vi "SaveLoadPreview-main.vi"(6 "error in":errorcluster, 10 "Prev-Save-Load":T1) -> (4 "error out 3":errorcluster)   [LabVIEW 2016, in "SaveLoad.lvlib"]
doc: "Takes a vi and saves or loads set values depending on which cluster value is chosen"
uses:
  SaveLoad.lvlib
  saveloadprev.ctl
  Beamline sections/High Energy End/High energy.lvlib
  Beamline sections/R30/R30.lvlib
  Beamline sections/Transmission/Transmission.lvlib
  Beamline sections/Low Energy End/Low energy.lvlib
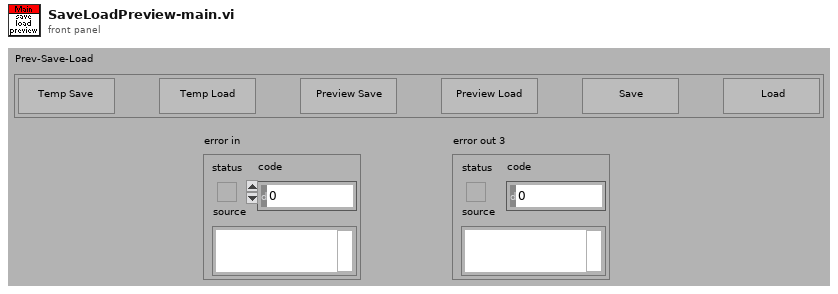
[diagram p1: front panel]
types:
  T1 = typedef "saveloadprev.ctl" = cluster{"Temp Save":bool, "Temp Load":bool, "Save":bool, "Load":bool, "Preview Save":bool, "Preview Load":bool}
  T2 = enum16{"open", "replace", "create", "open or create", "replace or create", "replace or create with confirmation"}
  T3 = typedef "prev-save-load-enum.ctl" = enum16{"Temp Save", "Temp Load", "Save", "Load", "Preview Save", "Preview Load"}
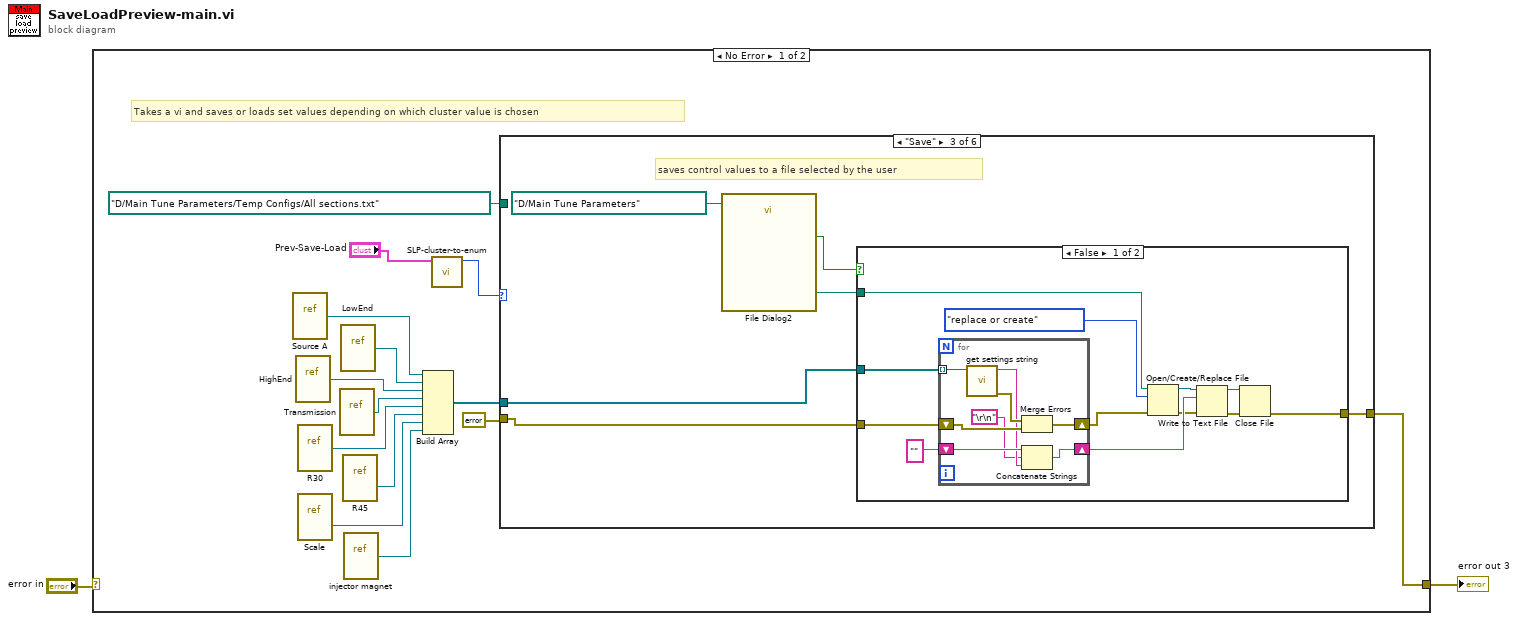
[diagram p0: block diagram]
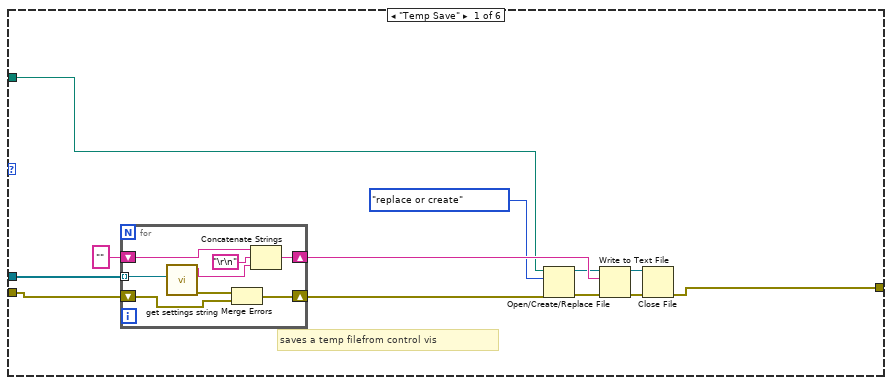
[diagram p2: hidden frame]
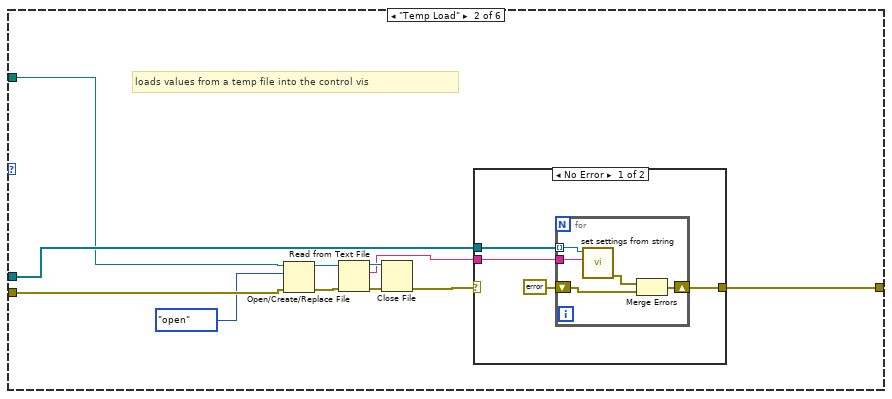
[diagram p3: hidden frame]
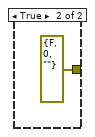
[diagram p5: hidden frame]
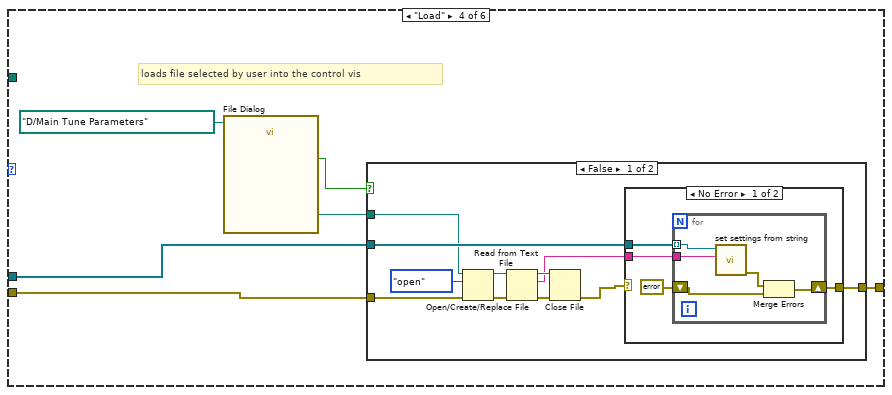
[diagram p6: hidden frame]
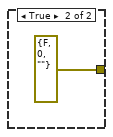
[diagram p8: hidden frame]
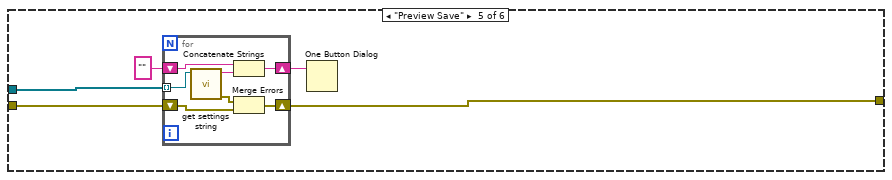
[diagram p9: hidden frame]
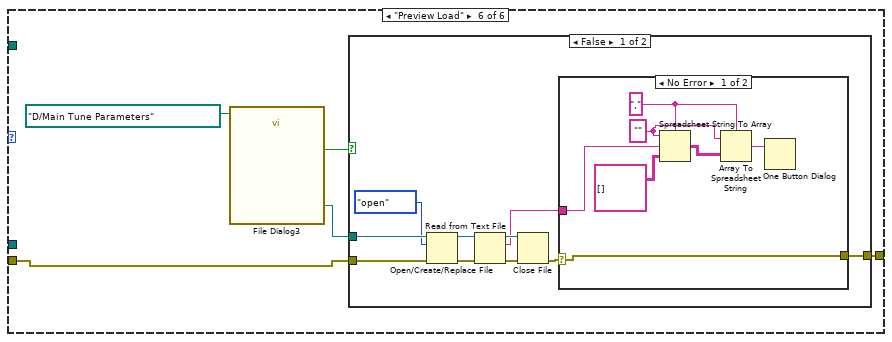
[diagram p10: hidden frame]
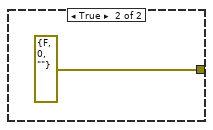
[diagram p12: hidden frame]
diagram:
  n1 = case shown="No Error" "error in" {
    selector: "error in" -> [_ w149]
    tunnel: [w16 w149] -> w2
    frame No Error {
      # "Takes a vi and saves or loads set values depending on which cluster value is chosen"
      n2 = vi-ref "Source A.vi"() -> (w10:refnum<vi>)
      n3 = vi-ref "HighEnd.vi"() -> (w14:refnum<vi>)
      n4 = vi-ref "R30.vi"() -> (w13:refnum<vi>)
      n5 = vi-ref "Scale.vi"() -> (w9:refnum<vi>)
      n6 = vi-ref "Transmission.vi"() -> (w15:refnum<vi>)
      n7 = vi-ref "LowEnd.vi"() -> (w11:refnum<vi>)
      n8 = vi-ref "R45.vi"() -> (w12:refnum<vi>)
      n9 = vi-ref "injector magnet.vi"() -> (w8:refnum<vi>)
      n10 = Build Array(w10, w11, w14, w15, w13, w12, w9, w8) -> (w7:refnum<vi>[])
      n11 = call "SLP-cluster-to-enum.vi"("Prev-Save-Load"="Prev-Save-Load") -> ("Prev-Save-Load enum"=w5:T3)  [unwired: 10 in]
      n12 = case shown="\"Save\"" w5 {
        tunnel: errorcluster {"status"=FALSE, "code"=0, "source"=""} ("error IO") -> [w17 w39 w62 w88 w113 w126]
        tunnel: [w24 w43 w61 w89 w114 w129] -> w16
        tunnel: w7 -> [w22 w45 w63 w90 w117 _]
        tunnel: path "D:/Main Tune Parameters/Temp Configs/All sections.txt" ("file path (use dialog)") -> [w20 w40 _ _ _ _]
        frame "Temp Save" {
          # "saves a temp filefrom control vis"
          n13 = for {
            shift-right: [w35] -> w28
            shift-left: "" -> [w34]
            tunnel: w22 -> [w33] mode=indexing
            shift-right: [w30] -> w23
            shift-left: w17 -> [w29]
            n14 = call "get settings string.vi"("VI in"=w33) -> ("error out"=w32:errorcluster, "Settings string"=w31:string)  [unwired: 9 in]
            n15 = Merge Errors(w32, w29) -> (w30:errorcluster)
            n16 = Concatenate Strings(w34, "\r\n", w31) -> (w35:string)
          }
          n17 = Open/Create/Replace File(file path (use dialog)=w20, error in=w23, operation (0:open)=T2."replace or create") -> (refnum out=w19:refnum<file>, error out=w21:errorcluster)  [unwired: 3 in, 1 out]
          n18 = Write to Text File(file (use dialog)=w19, text=w28, error in=w21) -> (refnum out=w26:refnum<file>, error out=w25:errorcluster)  [unwired: 1 in, 1 out]
          n19 = Close File(refnum=w26, error in=w25) -> (error out=w24:errorcluster)  [unwired: 1 out]
        }
        frame "Temp Load" {
          # "loads values from a temp file into the control vis"
          n20 = Open/Create/Replace File(file path (use dialog)=w40, error in=w39, operation (0:open)=T2."open") -> (refnum out=w41:refnum<file>, error out=w42:errorcluster)  [unwired: 3 in, 1 out]
          n21 = Read from Text File(file (use dialog)=w41, error in=w42) -> (refnum out=w47:refnum<file>, text=w44:string, error out=w46:errorcluster)  [unwired: 3 out]
          n22 = Close File(refnum=w47, error in=w46) -> (error out=w37:errorcluster)  [unwired: 1 out]
          n23 = case shown="No Error" w37 {
            selector: w37 -> [_ w57]
            tunnel: w45 -> [w51 _]
            tunnel: w44 -> [w50 _]
            tunnel: [w49 w57] -> w43
            frame No Error {
              n24 = for {
                tunnel: w51 -> [w55] mode=indexing
                tunnel: w50 -> [w56]
                shift-right: [w54] -> w49
                shift-left: errorcluster {"status"=FALSE, "code"=0, "source"=""} ("error IO") -> [w52]
                n25 = call "set settings from string.vi"("String"=w56, "VI in"=w55) -> ("error out"=w53:errorcluster)  [unwired: 9 in]
                n26 = Merge Errors(w53, w52) -> (w54:errorcluster)
              }
            }
            frame Error {
            }
          }
        }
        frame "Save" {
          # "saves control values to a file selected by the user"
          n27 = call "File Dialog2"("start path"=path "D:/Main Tune Parameters") -> ("selected path"=w59:path, "cancelled"=w58:bool)  [unwired: 11 in, 2 out]
          n28 = case shown="False" w58 {
            tunnel: w63 -> [w72 _]
            tunnel: w62 -> [w71 _]
            tunnel: [w64 errorcluster {"status"=FALSE, "code"=0, "source"=""} ("error out")] -> w61
            tunnel: w59 -> [w65 _]
            frame False {
              n29 = for {
                tunnel: w72 -> [w83] mode=indexing
                shift-right: [w81] -> w66
                shift-left: w71 -> [w80]
                shift-right: [w79] -> w70
                shift-left: "" -> [w78]
                n30 = call "get settings string.vi"("VI in"=w83) -> ("error out"=w82:errorcluster, "Settings string"=w77:string)  [unwired: 9 in]
                n31 = Merge Errors(w82, w80) -> (w81:errorcluster)
                n32 = Concatenate Strings(w78, "\r\n", w77) -> (w79:string)
              }
              n33 = Open/Create/Replace File(file path (use dialog)=w65, error in=w66, operation (0:open)=T2."replace or create") -> (refnum out=w68:refnum<file>, error out=w67:errorcluster)  [unwired: 1 in, 3 out]
              n34 = Write to Text File(file (use dialog)=w68, text=w70, error in=w67) -> (refnum out=w75:refnum<file>, error out=w74:errorcluster)  [unwired: 1 in, 1 out]
              n35 = Close File(refnum=w75, error in=w74) -> (error out=w64:errorcluster)  [unwired: 1 out]
            }
            frame True {
            }
          }
        }
        frame "Load" {
          # "loads file selected by user into the control vis"
          n36 = call "File Dialog"("start path"=path "D:/Main Tune Parameters") -> ("selected path"=w87:path, "cancelled"=w85:bool)  [unwired: 11 in, 2 out]
          n37 = case shown="False" w85 {
            tunnel: w90 -> [w99 _]
            tunnel: [w97 errorcluster {"status"=FALSE, "code"=0, "source"=""} ("error out")] -> w89
            tunnel: w88 -> [w96 _]
            tunnel: w87 -> [w92 _]
            frame False {
              n38 = Open/Create/Replace File(file path (use dialog)=w92, error in=w96, operation (0:open)=T2."open") -> (refnum out=w94:refnum<file>, error out=w95:errorcluster)  [unwired: 3 in, 1 out]
              n39 = Read from Text File(file (use dialog)=w94, error in=w95) -> (refnum out=w100:refnum<file>, text=w98:string, error out=w101:errorcluster)  [unwired: 3 out]
              n40 = Close File(refnum=w100, error in=w101) -> (error out=w91:errorcluster)  [unwired: 1 out]
              n41 = case shown="No Error" w91 {
                selector: w91 -> [_ w111]
                tunnel: w99 -> [w105 _]
                tunnel: w98 -> [w104 _]
                tunnel: [w103 w111] -> w97
                frame No Error {
                  n42 = for {
                    tunnel: w105 -> [w109] mode=indexing
                    tunnel: w104 -> [w110]
                    shift-right: [w108] -> w103
                    shift-left: errorcluster {"status"=FALSE, "code"=0, "source"=""} ("error IO") -> [w106]
                    n43 = call "set settings from string.vi"("String"=w110, "VI in"=w109) -> ("error out"=w107:errorcluster)  [unwired: 9 in]
                    n44 = Merge Errors(w107, w106) -> (w108:errorcluster)
                  }
                }
                frame Error {
                }
              }
            }
            frame True {
            }
          }
        }
        frame "Preview Save" {
          n45 = for {
            tunnel: w117 -> [w124] mode=indexing
            shift-right: [w122] -> w114
            shift-left: w113 -> [w121]
            shift-right: [w119] -> w115
            shift-left: "" -> [w118]
            n46 = call "get settings string.vi"("VI in"=w124) -> ("error out"=w123:errorcluster, "Settings string"=w120:string)  [unwired: 9 in]
            n47 = Concatenate Strings(w118, w120) -> (w119:string)
            n48 = Merge Errors(w123, w121) -> (w122:errorcluster)
          }
          n49 = One Button Dialog(message=w115) -> ()  [unwired: 1 in, 1 out]
        }
        frame "Preview Load" {
          n50 = call "File Dialog3"("start path"=path "D:/Main Tune Parameters") -> ("selected path"=w127:path, "cancelled"=w125:bool)  [unwired: 11 in, 2 out]
          n51 = case shown="False" w125 {
            tunnel: [w130 errorcluster {"status"=FALSE, "code"=0, "source"=""} ("error out")] -> w129
            tunnel: w127 -> [w136 _]
            tunnel: w126 -> [w132 _]
            frame False {
              n52 = Open/Create/Replace File(file path (use dialog)=w136, error in=w132, operation (0:open)=T2."open") -> (refnum out=w133:refnum<file>, error out=w134:errorcluster)  [unwired: 3 in, 1 out]
              n53 = Read from Text File(file (use dialog)=w133, error in=w134) -> (refnum out=w138:refnum<file>, text=w137:string, error out=w139:errorcluster)  [unwired: 3 out]
              n54 = Close File(refnum=w138, error in=w139) -> (error out=w131:errorcluster)  [unwired: 1 out]
              n55 = case shown="No Error" w131 {
                selector: w131 -> [w140 w147]
                tunnel: w137 -> [w145 _]
                tunnel: [w140 w147] -> w130
                frame No Error {
                  w142 = "," ("delimiter (Tab)")
                  w143 = "" ("format string")
                  n56 = Spreadsheet String To Array(delimiter (Tab)=w142, format string=w143, spreadsheet string=w145, array type (2D Dbl)=string[][] []) -> (array=w144:string[][])
                  n57 = Array To Spreadsheet String(delimiter (Tab)=w142, array=w144, 3:w143) -> (spreadsheet string=w141:string)
                  n58 = One Button Dialog(message=w141) -> ()  [unwired: 1 in, 1 out]
                }
                frame Error {
                }
              }
            }
            frame True {
            }
          }
        }
      }
    }
    frame Error {
    }
  }
  "error out 3" <- w2
